vi "Initialize Weather Station.vi"(8 "entrée d'erreur (pas d'erreur)":errorcluster) -> (0 "sortie d'erreur":errorcluster, 3 "refnum de fichier":refnum<file>, 5 "Données météo":T1)   [LabVIEW 2009]
doc: "Ce VI fait partie du projet Station météo. Le cluster de données météorologiques est créé ainsi qu'un fichier texte (méréo.txt). Un en-tête représentant le cluster de données météorologiques est écrit dans le fichier.\n\nEntrée : Entrée d'erreur\nSorties : Refnum de fichier, Cluster de données météorologiques, Sortie d'erreur."
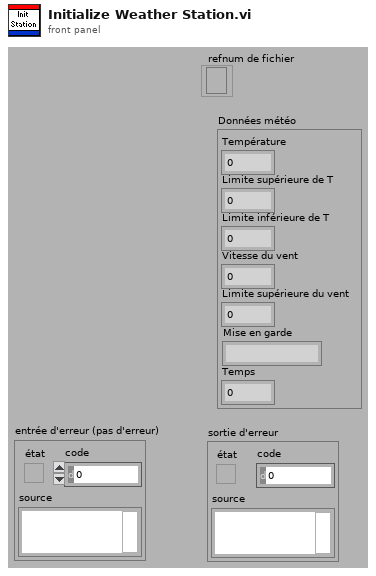
[diagram p1: front panel]
types:
  T1 = cluster{"Température":dbl, "Limite supérieure de T":dbl, "Limite inférieure de T":dbl, "Vitesse du vent":dbl, "Limite supérieure du vent":dbl, "Mise en garde":string, "Temps":dbl}
  T2 = enum16{"open", "replace", "create", "open or create", "replace or create", "replace or create with confirmation"}
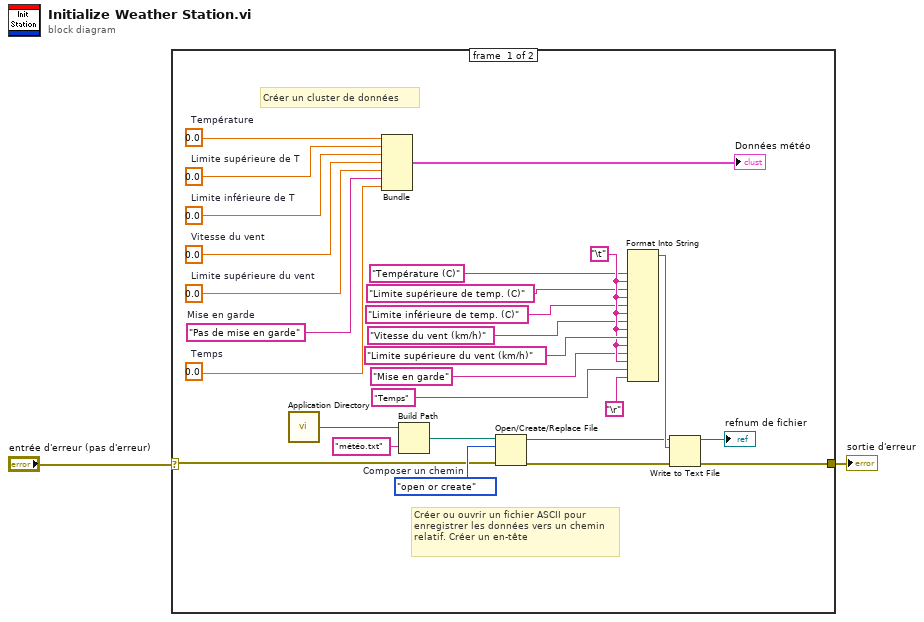
[diagram p0: block diagram]
diagram:
  n1 = case "Structure Condition" shown="Pas d'erreur" "entrée d'erreur (pas d'erreur)" {
    selector: "entrée d'erreur (pas d'erreur)" -> [w4 w30]
    tunnel: [w28 w30] -> w2
    frame #0 {
      w12 = 0.0  # Temps
      w11 = 0.0  # Limite supérieure du vent
      w10 = 0.0  # Vitesse du vent
      w5 = 0.0  # Limite inférieure de T
      w6 = 0.0  # Limite supérieure de T
      w7 = 0.0  # Température
      w22 = "\t"
      w9 = "Pas de mise en garde"  # Mise en garde
      # "Créer ou ouvrir un fichier ASCII pour enregistrer les données vers un chemin relatif. Créer un en-tête"
      # "Créer un cluster de données"
      n2 = call <vilib>:"Application Directory.vi"() -> ("Application Directory"=w3:path)
      n3 = Bundle ("Assembler")("Température"=w7, "Limite supérieure de T"=w6, "Limite inférieure de T"=w5, "Vitesse du vent"=w10, "Limite supérieure du vent"=w11, "Mise en garde"=w9, "Temps"=w12) -> (→"Données météo":T1)  [unwired: 1 in]
      n4 = Build Path "Composer un chemin"(base path=w3, name or relative path="météo.txt") -> (appended path=w14:path)
      n5 = Open/Create/Replace File ("Ouvrir/Créer/Remplacer un fichier")(file path (use dialog)=w14, error in=w4, operation (0:open)=T2."open or create") -> (refnum out=w25:refnum<file>, error out=w27:errorcluster)  [unwired: 3 in, 1 out]
      n6 = Format Into String ("Formater en chaîne")("Température (C)", w22, "Limite supérieure de temp. (C)", w22, "Limite inférieure de temp. (C)", w22, "Vitesse du vent (km/h)", w22, "Limite supérieure du vent (km/h)", w22, "Mise en garde", w22, "Temps", "\r") -> (resulting string=w29:string)  [unwired: 3 in, 1 out]
      n7 = Write to Text File ("Écrire dans un fichier texte")(file (use dialog)=w25, text=w29, error in=w27) -> (refnum out=→"refnum de fichier":refnum<file>, error out=w28:errorcluster)  [unwired: 1 in, 1 out]
    }
    frame #1 {
    }
  }
  "sortie d'erreur" <- w2
